vi "Write Topic Registry.vi"(8 "error in":errorcluster, 10 "Topic Registry":T1[](array[typedef]), 11 "Broker in":refnum<class "Broker.lvclass">) -> (0 "error out":errorcluster, 3 "Broker out":refnum<class "Broker.lvclass">)   [LabVIEW 2014, in "Broker.lvclass"]
uses:
  Broker.lvclass
  Controls/Topic Ref.ctl
  Broker.lvclass/Broker.ctl
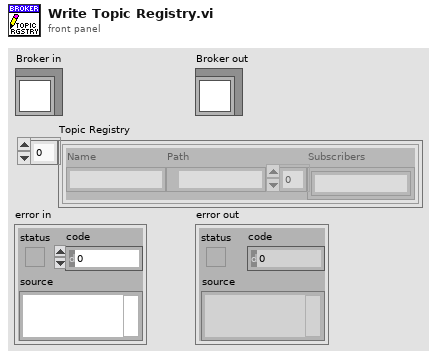
[diagram p1: front panel]
types:
  T1 = typedef "Topic Ref.ctl" = cluster{"Name":string, "Path":path, "Subscribers":string[]}
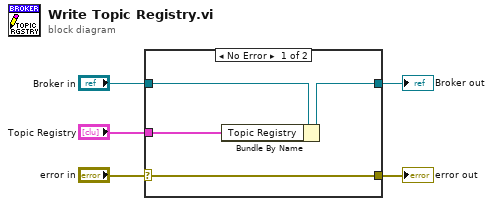
[diagram p0: block diagram]
diagram:
  n1 = case shown="No Error" "error in" {
    selector: "error in" -> [w9 w10]
    tunnel: [w9 w10] -> w4
    tunnel: [w7 w11] -> w2
    tunnel: "Broker in" -> [w8 w11]
    tunnel: "Topic Registry" -> [w6 _]
    frame No Error {
      n2 = Bundle By Name(cluster=w8, "Topic Registry"=w6) -> (w7:refnum<class "Broker.lvclass">)
    }
    frame Error {
    }
  }
  "error out" <- w4
  "Broker out" <- w2
